vi "Stop Core.vi"(10 "final error code":i32, 11 "Measurement Generator in":refnum<class "Measurement Generator.lvclass">) -> (3 "Measurement Generator out":refnum<class "Measurement Generator.lvclass">)   [LabVIEW 2020, in "Measurement Generator.lvclass"]
doc: "(<B>Filename</B>: Actor Framework.lvlib:Actor.lvclass:Stop Core.vi)\n\nDefines what the actor does before it stops. Use the <B>final error code</B> input to determine whether the actor shut down in response to an error.\n\nBy default, this method passes the Stop message along to all auto-stop nested actors. A descendant class may override this method to define additional behavior, such as shutting down any processes the actor initiated in its override of the Actor Core method."
uses:
  Measurement Generator.lvclass
  <vilib>/ActorFramework/Actor/Actor.lvclass
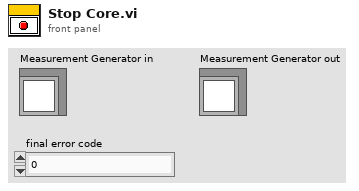
[diagram p1: front panel]
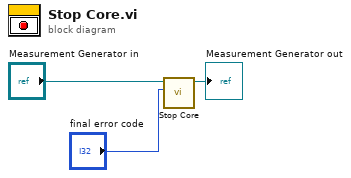
[diagram p0: block diagram]
diagram:
  n1 = call-parent "Stop Core.vi"("final error code"="final error code", "Actor in"="Measurement Generator in") -> ("Actor out"=→"Measurement Generator out":refnum<class "Measurement Generator.lvclass">)  [unwired: 9 in]
